vi "demo_hub_geti.vi"() -> ()   [LabVIEW 2017]
panel:
  in  "停止":bool
  out "数字 4":i32
  out "数字 3":i32
  out "数字 2":i32
  out "数字":i32
  in  "name":string="hub1"
  in  "ip":string="192.168.1.123"
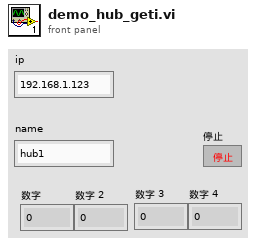
[diagram p1: front panel]
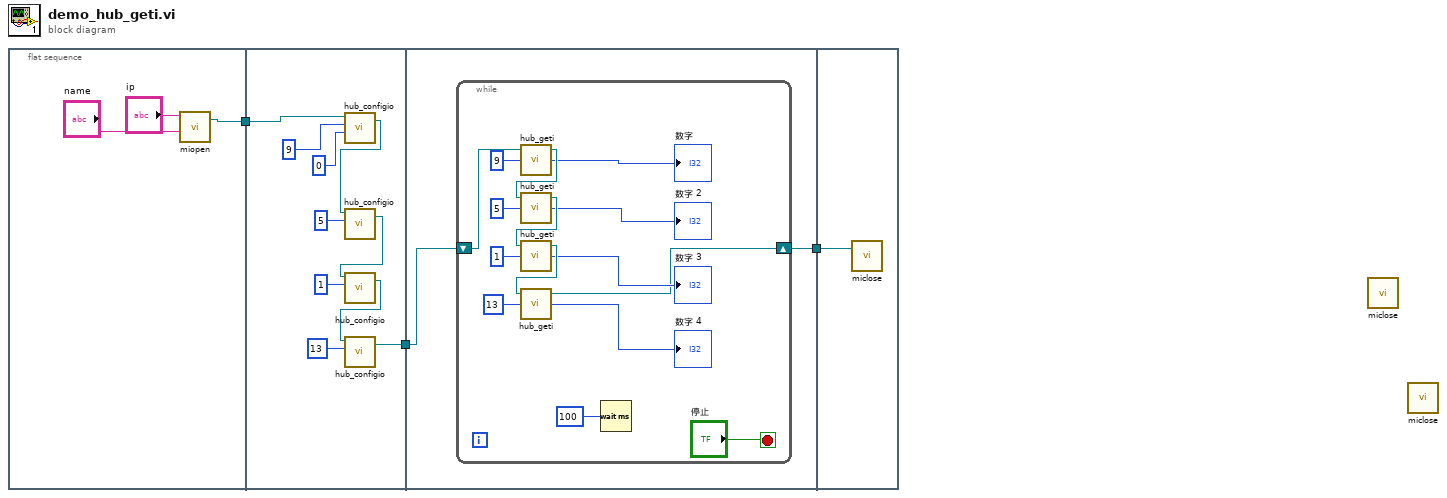
[diagram p0: block diagram]
diagram:
  n1 = flat-sequence {
    tunnel: [w4] -> w1
    tunnel: [w8] -> w3
    tunnel: w1 -> [w7]
    tunnel: w3 -> [w18]
    tunnel: [w17] -> w2
    tunnel: w2 -> [w34]
    frame #0 {
      n2 = call "miopen.vi"("name"="name", "ip"="ip") -> ("VISA资源名称输出"=w4:refnum<visa-resource-name>)  [unwired: 2 in, 1 out]
    }
    frame #1 {
      n3 = call "hub_configio.vi"("输入 2"=0, "输入 1"=9, "VISA资源名称"=w7) -> ("VISA资源名称输出"=w15:refnum<visa-resource-name>)  [unwired: 1 in, 1 out]
      n4 = call "hub_configio.vi"("输入 1"=5, "VISA资源名称"=w15) -> ("VISA资源名称输出"=w14:refnum<visa-resource-name>)  [unwired: 2 in, 1 out]
      n5 = call "hub_configio.vi"("输入 1"=1, "VISA资源名称"=w14) -> ("VISA资源名称输出"=w13:refnum<visa-resource-name>)  [unwired: 2 in, 1 out]
      n6 = call "hub_configio.vi"("输入 1"=13, "VISA资源名称"=w13) -> ("VISA资源名称输出"=w8:refnum<visa-resource-name>)  [unwired: 2 in, 1 out]
    }
    frame #2 {
      n7 = while {
        shift-right: [w21] -> w17
        shift-left: w18 -> [w33]
        stop <- "停止" stop-if-true
        n8 = call "hub_geti.vi"("输入 1"=9, "VISA资源名称"=w33) -> ("数字"=→"数字":i32, "VISA资源名称输出"=w32:refnum<visa-resource-name>)  [unwired: 1 in, 1 out]
        n9 = call "hub_geti.vi"("输入 1"=5, "VISA资源名称"=w32) -> ("数字"=→"数字 2":i32, "VISA资源名称输出"=w31:refnum<visa-resource-name>)  [unwired: 1 in, 1 out]
        n10 = call "hub_geti.vi"("输入 1"=1, "VISA资源名称"=w31) -> ("数字"=→"数字 3":i32, "VISA资源名称输出"=w30:refnum<visa-resource-name>)  [unwired: 1 in, 1 out]
        n11 = call "hub_geti.vi"("输入 1"=13, "VISA资源名称"=w30) -> ("数字"=→"数字 4":i32, "VISA资源名称输出"=w21:refnum<visa-resource-name>)  [unwired: 1 in, 1 out]
        n12 = Wait (ms)(milliseconds to wait=u32 100 ("等待时间（毫秒）")) -> ()  [unwired: 1 out]
      }
    }
    frame #3 {
      n13 = call "miclose.vi"("VISA资源名称"=w34) -> ()  [unwired: 1 in, 1 out]
    }
  }
  n14 = call "miclose.vi"() -> ()  [unwired: 2 in, 1 out]
  n15 = call "miclose.vi"() -> ()  [unwired: 2 in, 1 out]
